vi "Stop.vi"(8 "error in (no error)":errorcluster, 10 "Message in":refnum<class "StopMessage.lvclass">, 11 "Thorcam in":refnum<class "Thorcam.lvclass">) -> (0 "error out":errorcluster, 3 "Thorcam out":refnum<class "Thorcam.lvclass">)   [LabVIEW 2012, in "Thorcam.lvclass"]
doc: "This member function is called when the statemachine in the run.vi receives an 'stop' command. It relays the message to all observers of the component.\n\nOverride this member function in your derived class if you need additional stop functionality (but don't forget to call the parent method)."
uses:
  Thorcam.lvclass
  <vilib>/Distrio/Murmex/Murmex/Murmex.lvclass
  <vilib>/Distrio/Murmex/StopMessage/StopMessage.lvclass
panel:
  # "This method is called when the STOP\ntrigger is sent. \n\nOverride this method when your component needs to\nrespond to this trigger. \n\nCall parent for proper implementation"
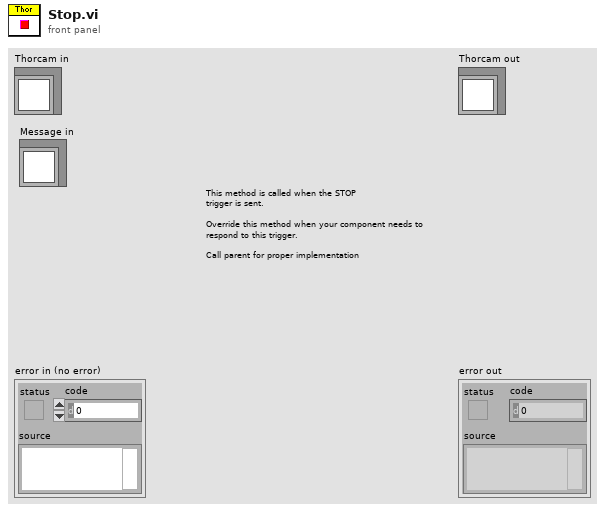
[diagram p1: front panel]
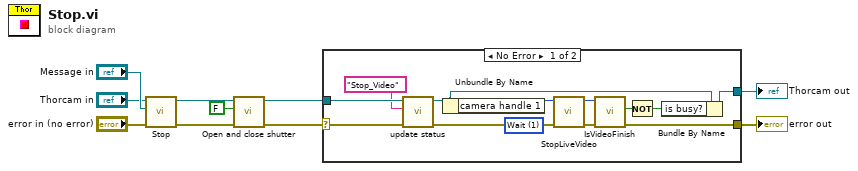
[diagram p0: block diagram]
diagram:
  n1 = call-parent "Stop.vi"("error in (no error)"="error in (no error)", "Message in"="Message in", "Murmex in"="Thorcam in") -> ("error out"=w7:errorcluster, "Murmex out"=w3:refnum<class "Thorcam.lvclass">)  [unwired: 7 in]
  n2 = call-dynamic "Open and close shutter.vi"("error in (no error)"=w7, "Open?"=FALSE, "Thorcam in"=w3) -> ("error out"=w4:errorcluster, "Thorcam out"=w2:refnum<class "Thorcam.lvclass">)  [unwired: 7 in]
  n3 = case shown="No Error" w4 {
    selector: w4 -> [w16 w24]
    tunnel: w2 -> [w14 w25]
    tunnel: [w22 w25] -> w6
    tunnel: [w19 w24] -> w5
    frame No Error {
      w11 = 1 items=["Dont't Wait"=0, "Wait"=1, "Force Video Stop"=16384] ("Wait")
      n4 = call-dynamic "update status.vi"("error in (no error)"=w16, "status in"="Stop_Video", "Thorcam in"=w14) -> ("error out"=w15:errorcluster, "Thorcam out"=w13:refnum<class "Thorcam.lvclass">)  [unwired: 7 in]
      n5 = Unbundle By Name(w13) -> ("camera handle 1"=w23:u32)
      n6 = call <instrlib>:"StopLiveVideo.vi"("error in"=w15, "Wait"=w11, "Camera Handle In"=w23) -> ("error out"=w20:errorcluster, "Camera Handle Out"=w21:u32)  [unwired: 7 in]
      n7 = call <instrlib>:"IsVideoFinish.vi"("error in"=w20, "Camera Handle In"=w21) -> ("error out"=w19:errorcluster, "Video Finish"=w18:bool)  [unwired: 7 in, 1 out]
      n8 = Not(x=w18) -> (.not. x?=w17:bool)
      n9 = Bundle By Name(cluster=w13, "is busy?"=w17) -> (w22:refnum<class "Thorcam.lvclass">)
    }
    frame Error {
    }
  }
  "error out" <- w5
  "Thorcam out" <- w6
